vi "get Data.vi"(11 "RAM in":refnum<class "RAM.lvclass">) -> (3 "Data":u8[](array[numeric]))   [LabVIEW 2021, in "RAM.lvclass"]
uses:
  RAM.lvclass
  RAM.lvclass/RAM.ctl
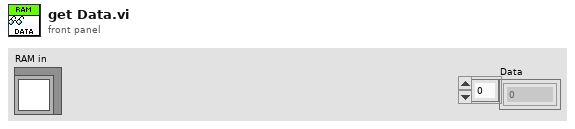
[diagram p1: front panel]
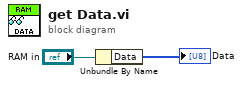
[diagram p0: block diagram]
diagram:
  n1 = Unbundle By Name("RAM in") -> ("Data"=→"Data":u8[])
